vi "Test.vi"   [LabVIEW 2020, in "Sequencer.lvclass"]
uses:
  Sequencer.lvclass
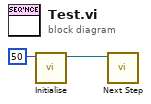
[diagram p0: block diagram]
diagram:
  n1 = call "Initialise.vi"("Max Steps (10)"=50 ("Max Steps (100)")) -> ("Sequencer out"=w1:refnum<class "Sequencer.lvclass">)  [unwired: 9 in, 1 out]
  n2 = call "Next Step.vi"("Sequencer in"=w1) -> ()  [unwired: 6 in, 5 out]
